vi "Build date time subfolder.vi"() -> (3 "User folder appended with daily folder":path)   [LabVIEW 2020]
uses:
  Global Variables/General Globals.vi
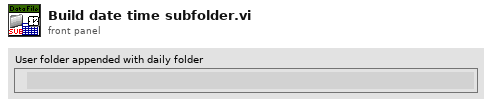
[diagram p1: front panel]
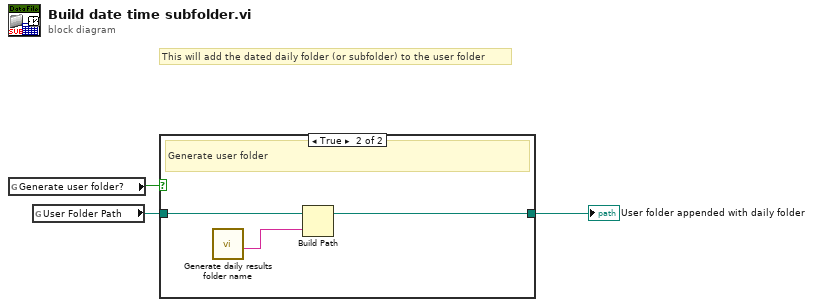
[diagram p0: block diagram]
diagram:
  # "This will add the dated daily folder (or subfolder) to the user folder"
  n1 = global read "General Globals.vi" "Generate user folder?"() -> (w2:bool)
  n2 = global read "General Globals.vi" "User Folder Path"() -> (w1:path)
  n3 = case shown="True" w2 {
    tunnel: w1 -> [w4 w7]
    tunnel: [w4 w6] -> w3
    frame False {
      # "Do not generate user folder"
    }
    frame True {
      # "Generate user folder"
      n4 = call "Generate daily results folder name.vi"() -> ("Generated daily folder name"=w5:string)  [unwired: 11 in]
      n5 = Build Path(base path=w7, name or relative path=w5) -> (appended path=w6:path)
    }
  }
  "User folder appended with daily folder" <- w3
